vi "examen2_1.vi"() -> ()   [LabVIEW 2020]
panel:
  out "String":string
  in  "Tab Control":enum32{"servicio", "mantenimiento"}(tab)=enum."mantenimiento"
  in  "COFFEE":bool
  in  "COLD DRINK":bool
  in  "CANDIES":bool
  in  "SNACKS":bool
  in  "$20":bool
  in  "$10":bool
  out "$ INGRESADA":dbl
  in  "INICILIZAR":bool
  out "$ DEVOLVER":dbl
  out "$ FALTANTE":dbl
  in  "CANCELAR":bool
  out "v. $10":dbl
  out "v. $20":dbl
  in  "in. snack":dbl=4.0
  in  "in. coffee":dbl=4.0
  in  "in. cold drink":dbl=4.0
  in  "in. candies":dbl=4.0
  # "VALOR IN $ 10"
  # "VALOR IN $ 20"
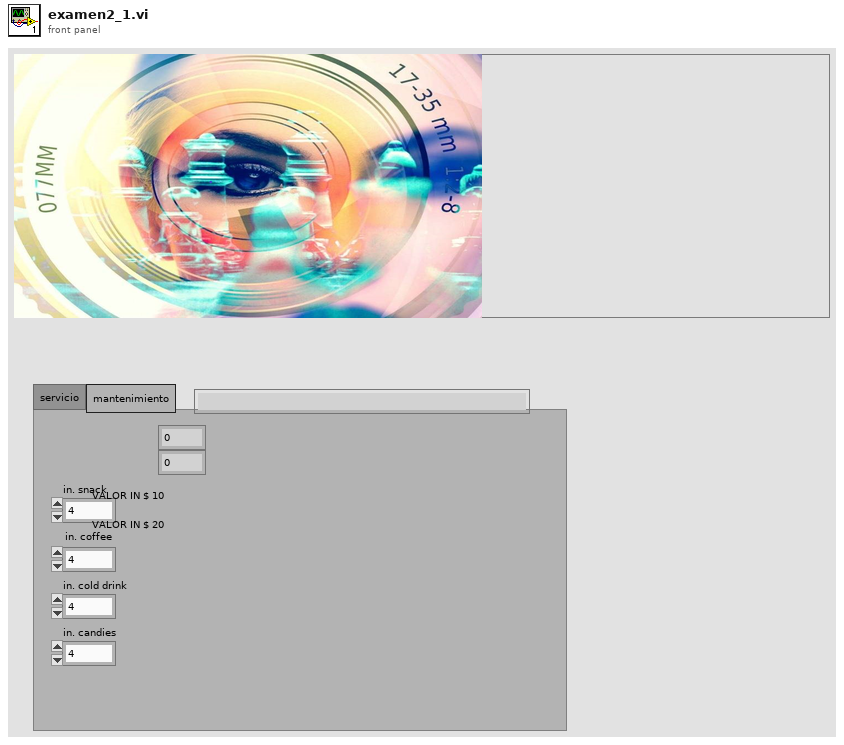
[diagram p1: front panel]
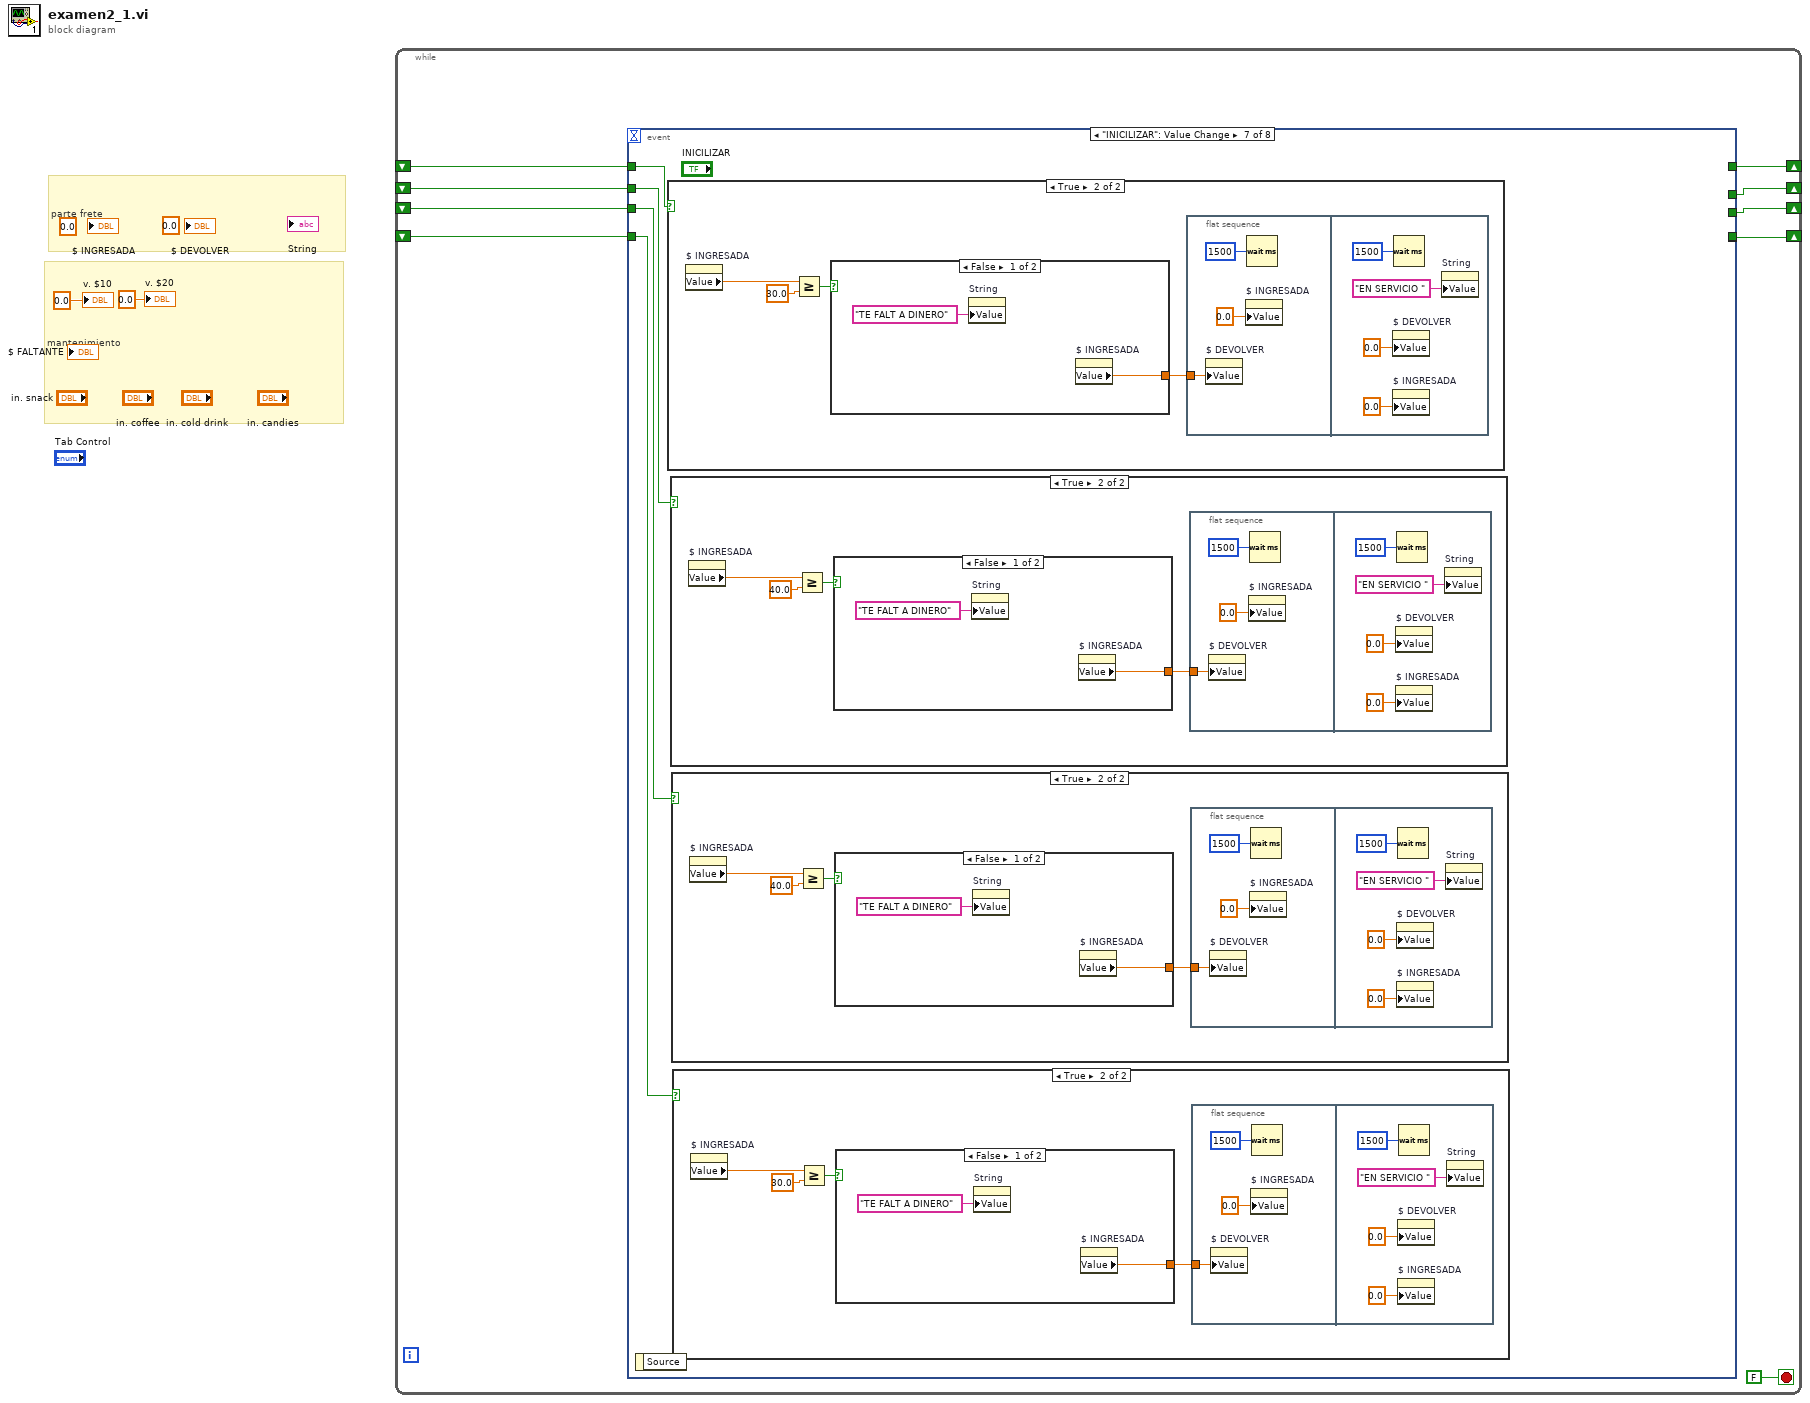
[diagram p0: block diagram]
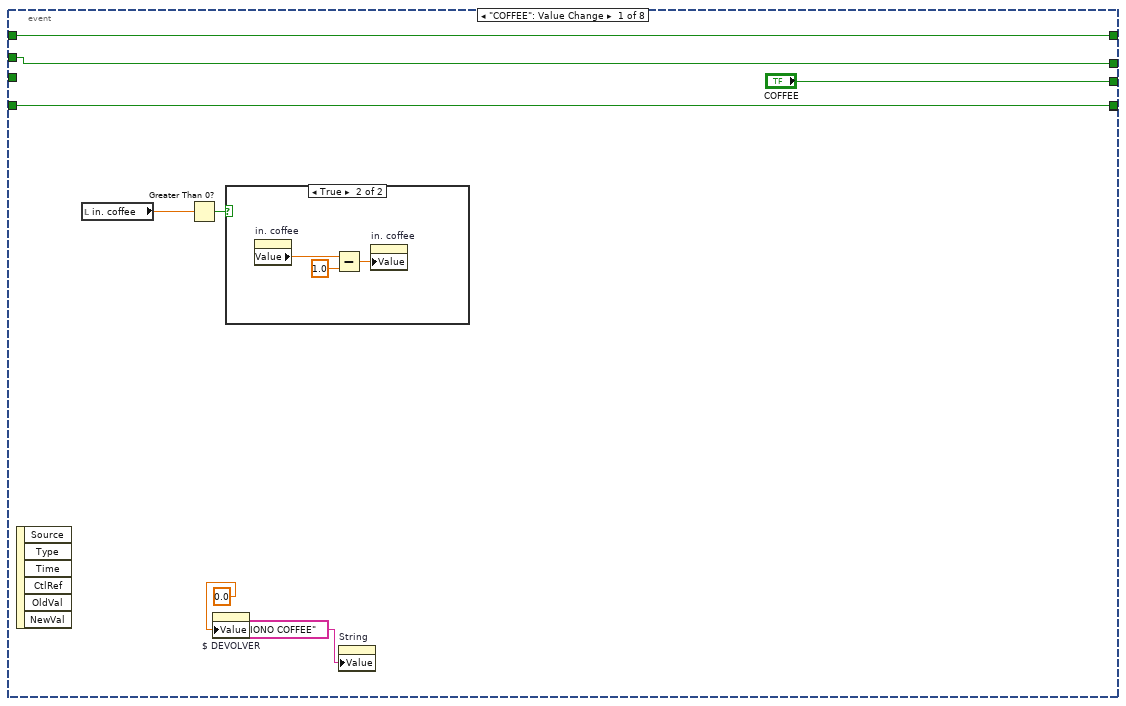
[diagram p2: hidden frame]
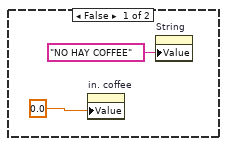
[diagram p3: hidden frame]
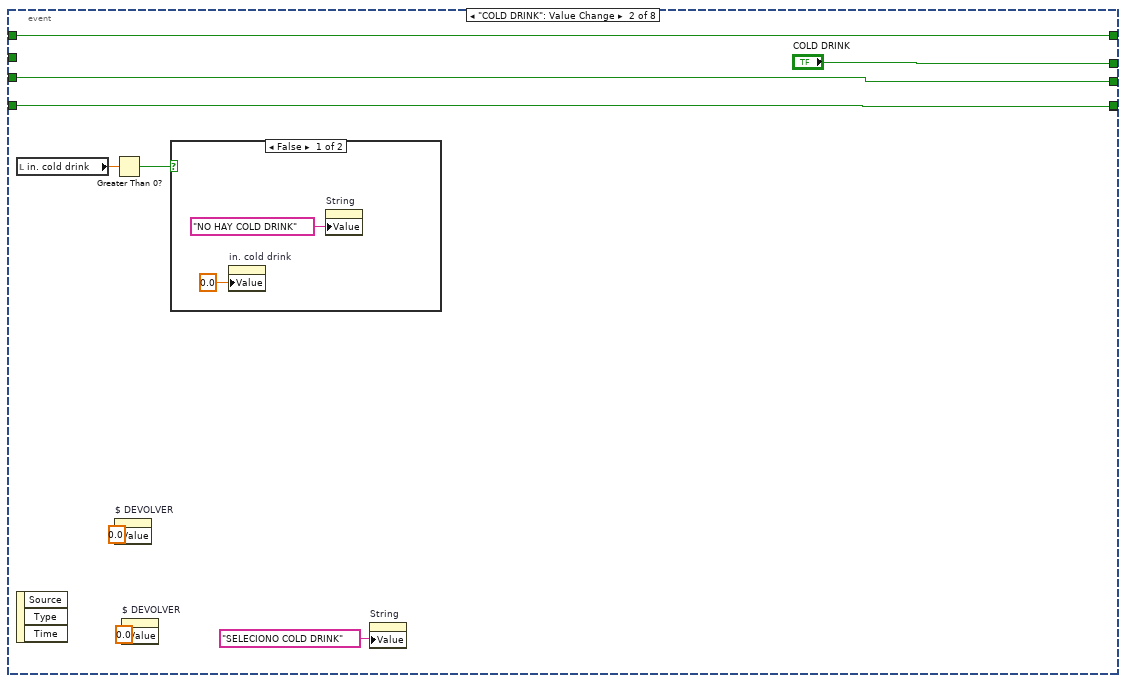
[diagram p4: hidden frame]
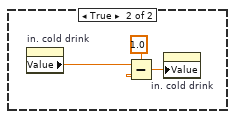
[diagram p5: hidden frame]
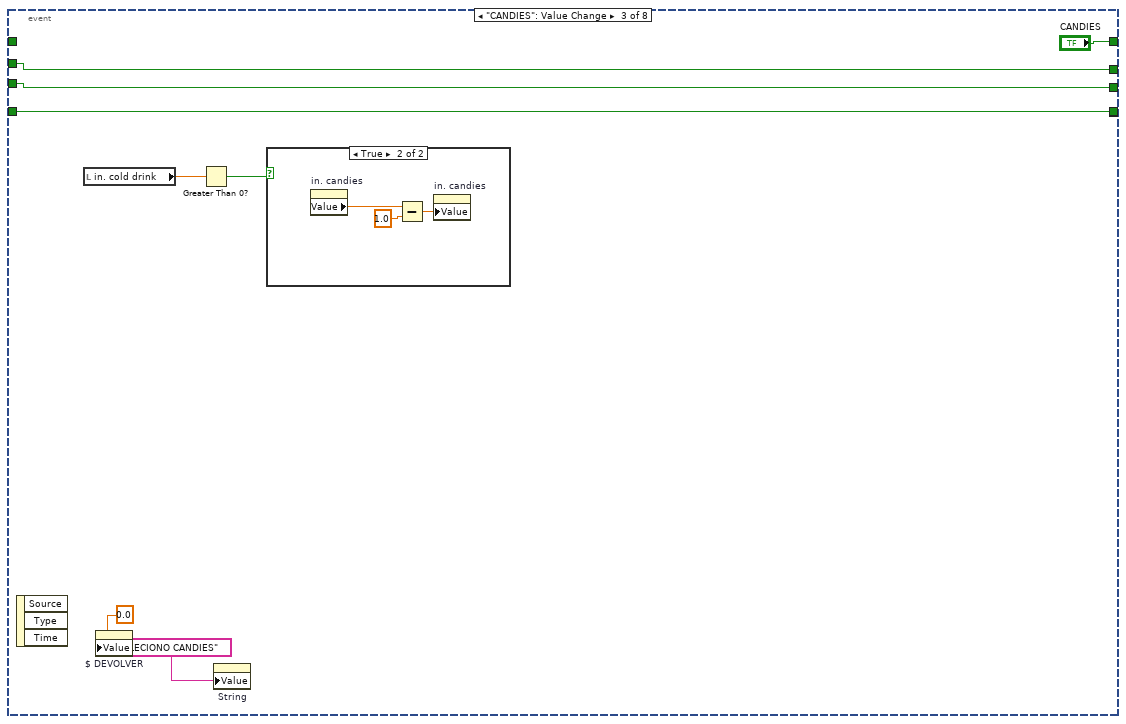
[diagram p6: hidden frame]
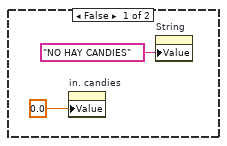
[diagram p7: hidden frame]
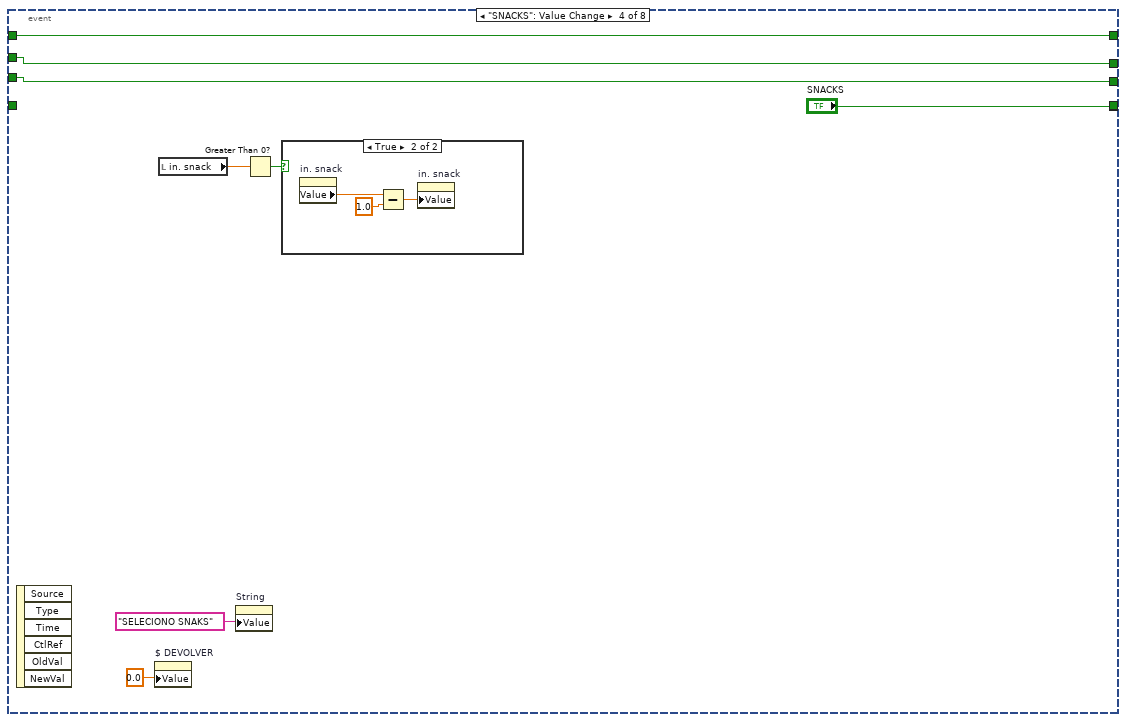
[diagram p8: hidden frame]
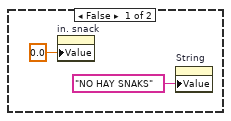
[diagram p9: hidden frame]
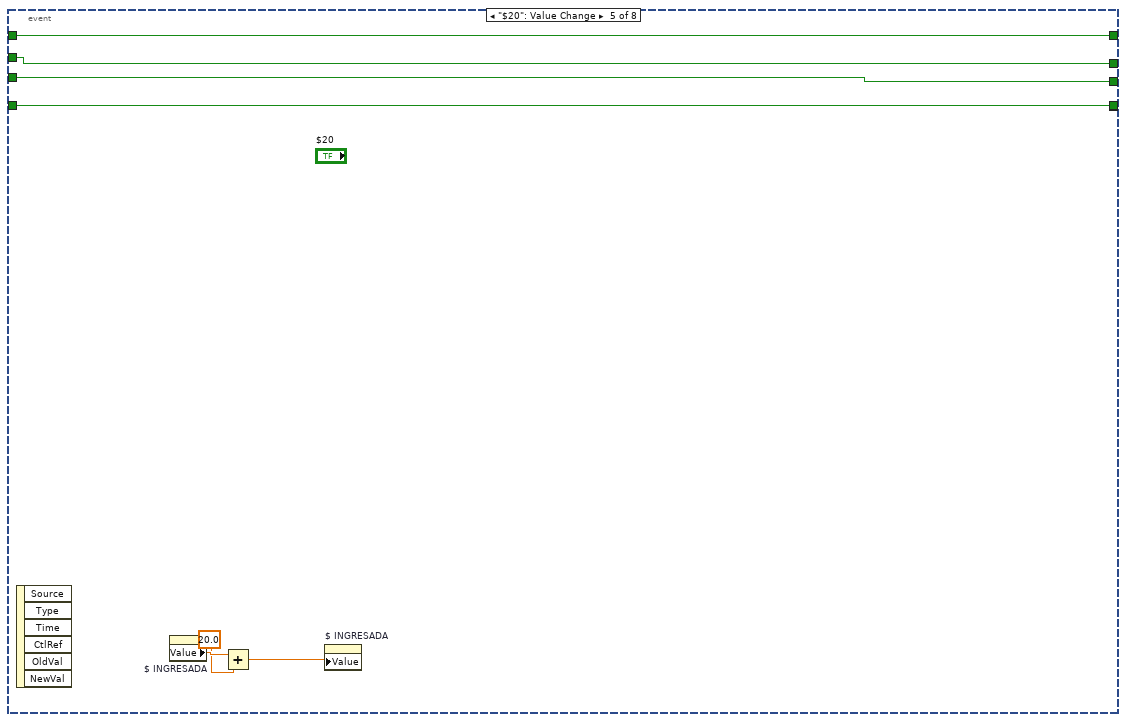
[diagram p10: hidden frame]
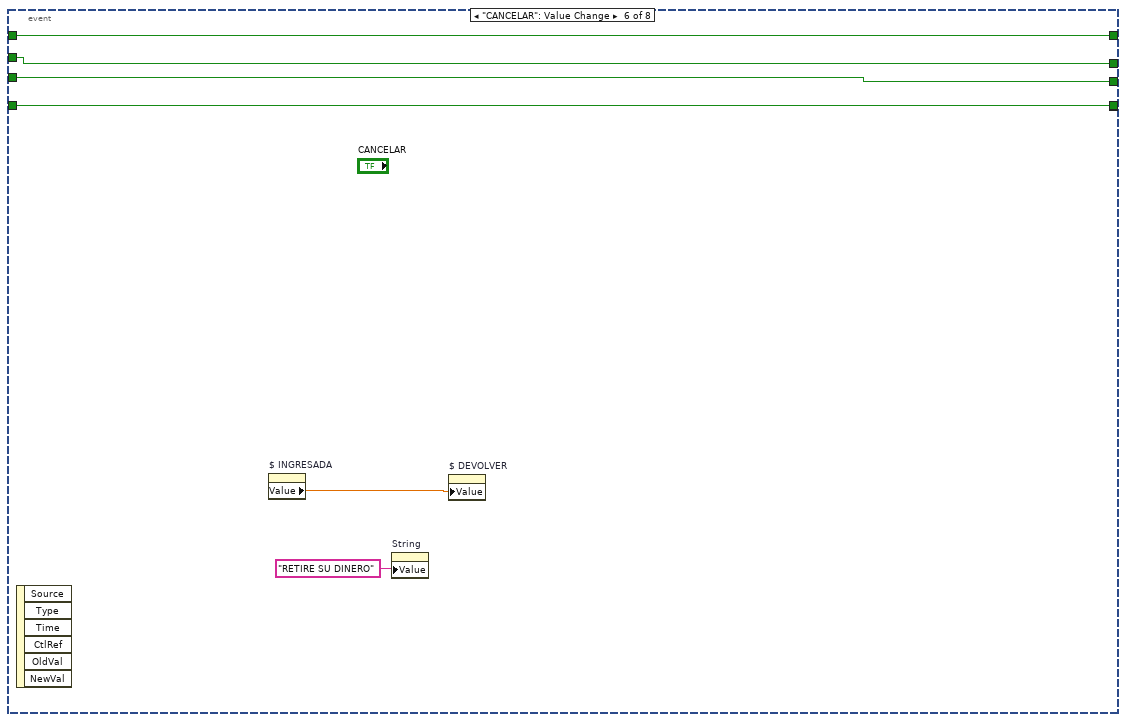
[diagram p11: hidden frame]
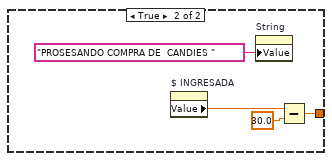
[diagram p13: hidden frame]
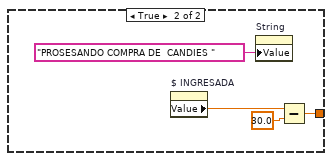
[diagram p15: hidden frame]
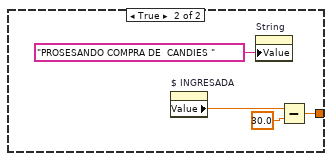
[diagram p17: hidden frame]
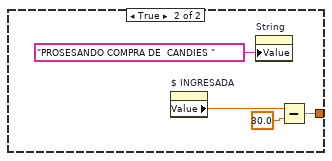
[diagram p19: hidden frame]
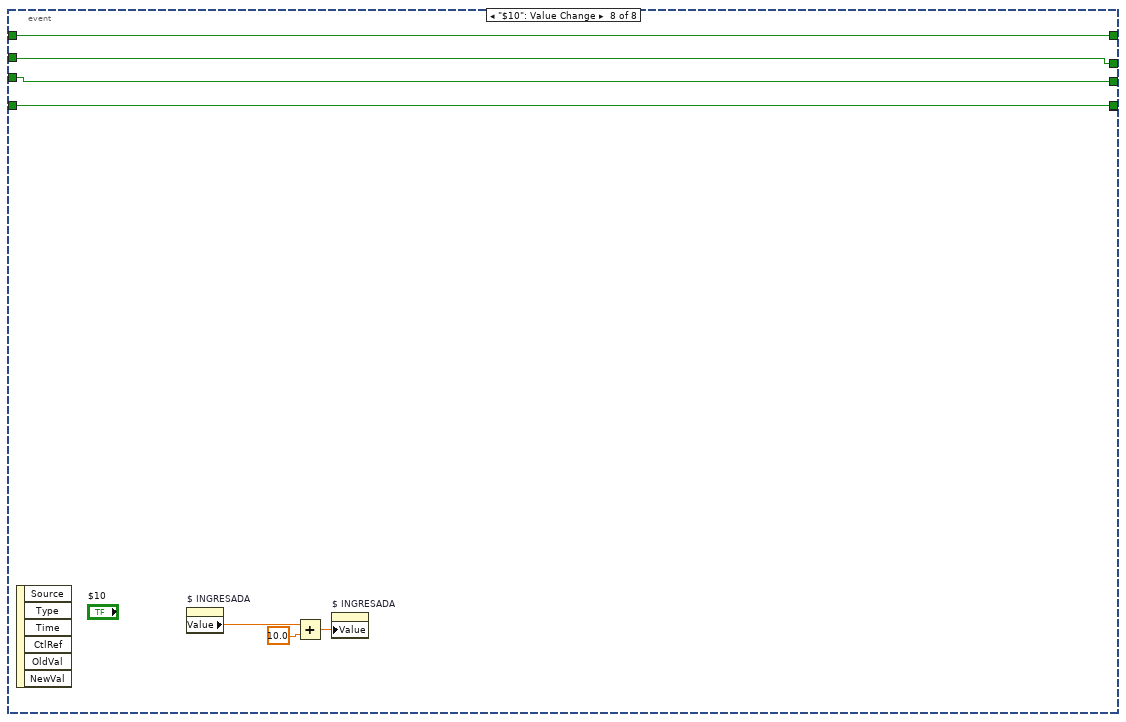
[diagram p20: hidden frame]
diagram:
  # "parte frete"
  # "mantenimiento"
  n1 = while {
    shift-right: [w12] -> _
    shift-left: _ -> [w11]
    shift-right: [w10] -> _
    shift-left: _ -> [w9]
    shift-right: [w8] -> _
    shift-left: _ -> [w7]
    shift-right: [w6] -> _
    shift-left: _ -> [w5]
    stop <- FALSE stop-if-true
    n2 = event shown="[6] \"INICILIZAR\": Value Change" {
      selector: _ -> [_ _ _ _ _ _ _ _]
      dyn-events: _ -> [_ _ _ _ _ _ _ _]
      timeout: _ -> [_ _ _ _ _ _ _ _]
      tunnel: [w19 "COLD DRINK" w46 w59 w70 w76 _ w155] -> w12
      tunnel: w11 -> [w19 _ w46 w59 w70 w76 w80 w155]
      tunnel: [w16 w29 "CANDIES" w58 w69 _ _ w154] -> w10
      tunnel: w9 -> [w16 w29 _ w58 w69 w77 w83 w154]
      tunnel: ["COFFEE" w28 w42 w57 w68 w74 _ w153] -> w8
      tunnel: w7 -> [_ w28 w42 w57 w68 w74 w81 w153]
      tunnel: [w14 w27 w41 "SNACKS" w67 _ _ w152] -> w6
      tunnel: w5 -> [w14 w27 w41 _ w67 w75 w82 w152]
      tunnel: [_ _ _ _ _ w77 _ _] -> _
      tunnel: [_ _ _ _ _ w75 _ _] -> _
      event "COFFEE": Value Change {
        n3 = event-data() -> ()  [unwired: 1 in, 6 out]
        n4 = local read "in. coffee"() -> (w18:dbl)
        n5 = Greater Than 0?(x=w18) -> (x > 0?=w17:bool)
        n6 = property on="$ DEVOLVER" class="DigNum (strict)"("Value"=0.0 ("$ DEVOLVER")) -> ()  [unwired: 2 in, 2 out]
        n7 = case shown="True" w17 {
          frame False {
            n8 = property on="in. coffee" class="DigNum (strict)"("Value"=0.0 ("in. cold drink")) -> ()  [unwired: 2 in, 2 out]
            n9 = property on="String" class="Str"("Value"="NO HAY COFFEE" ("String")) -> ()  [unwired: 2 in, 2 out]
          }
          frame True {
            n10 = property on="in. coffee" class="DigNum (strict)"() -> ("Value"=w26:dbl)  [unwired: 2 in, 2 out]
            n11 = Subtract(x=w26, y=1.0) -> (x-y=w25:dbl)
            n12 = property on="in. coffee" class="DigNum (strict)"("Value"=w25) -> ()  [unwired: 2 in, 2 out]
          }
        }
        n13 = property on="String" class="Str"("Value"="SELECIONO COFFEE" ("String")) -> ()  [unwired: 2 in, 2 out]
      }
      event "COLD DRINK": Value Change {
        n14 = local read "in. cold drink"() -> (w33:dbl)
        n15 = event-data() -> ()  [unwired: 1 in, 3 out]
        n16 = Greater Than 0?(x=w33) -> (x > 0?=w32:bool)
        n17 = property on="$ DEVOLVER" class="DigNum (strict)"("Value"=0.0 ("$ DEVOLVER")) -> ()  [unwired: 2 in, 2 out]
        n18 = property on="$ DEVOLVER" class="DigNum (strict)"("Value"=0.0 ("$ DEVOLVER")) -> ()  [unwired: 2 in, 2 out]
        n19 = case shown="False" w32 {
          frame False {
            n20 = property on="in. cold drink" class="DigNum (strict)"("Value"=0.0 ("in. cold drink")) -> ()  [unwired: 2 in, 2 out]
            n21 = property on="String" class="Str"("Value"="NO HAY COLD DRINK" ("String")) -> ()  [unwired: 2 in, 2 out]
          }
          frame True {
            n22 = property on="in. cold drink" class="DigNum (strict)"() -> ("Value"=w40:dbl)  [unwired: 2 in, 2 out]
            n23 = Subtract(x=w40, y=1.0) -> (x-y=w39:dbl)
            n24 = property on="in. cold drink" class="DigNum (strict)"("Value"=w39) -> ()  [unwired: 2 in, 2 out]
          }
        }
        n25 = property on="String" class="Str"("Value"="SELECIONO COLD DRINK" ("String")) -> ()  [unwired: 2 in, 2 out]
      }
      event "CANDIES": Value Change {
        n26 = event-data() -> ()  [unwired: 1 in, 3 out]
        n27 = local read "in. cold drink"() -> (w45:dbl)
        n28 = property on="$ DEVOLVER" class="DigNum (strict)"("Value"=0.0 ("$ DEVOLVER")) -> ()  [unwired: 2 in, 2 out]
        n29 = Greater Than 0?(x=w45) -> (x > 0?=w44:bool)
        n30 = property on="String" class="Str"("Value"="SELECIONO CANDIES" ("String")) -> ()  [unwired: 2 in, 2 out]
        n31 = case shown="True" w44 {
          frame False {
            n32 = property on="in. candies" class="DigNum (strict)"("Value"=0.0 ("in. cold drink")) -> ()  [unwired: 2 in, 2 out]
            n33 = property on="String" class="Str"("Value"="NO HAY CANDIES" ("String")) -> ()  [unwired: 2 in, 2 out]
          }
          frame True {
            n34 = property on="in. candies" class="DigNum (strict)"() -> ("Value"=w53:dbl)  [unwired: 2 in, 2 out]
            n35 = Subtract(x=w53, y=1.0) -> (x-y=w52:dbl)
            n36 = property on="in. candies" class="DigNum (strict)"("Value"=w52) -> ()  [unwired: 2 in, 2 out]
          }
        }
      }
      event "SNACKS": Value Change {
        n37 = event-data() -> ()  [unwired: 1 in, 6 out]
        n38 = property on="$ DEVOLVER" class="DigNum (strict)"("Value"=0.0 ("$ DEVOLVER")) -> ()  [unwired: 2 in, 2 out]
        n39 = local read "in. snack"() -> (w55:dbl)
        n40 = property on="String" class="Str"("Value"="SELECIONO SNAKS" ("String")) -> ()  [unwired: 2 in, 2 out]
        n41 = Greater Than 0?(x=w55) -> (x > 0?=w54:bool)
        n42 = case shown="True" w54 {
          frame False {
            n43 = property on="in. snack" class="DigNum (strict)"("Value"=0.0 ("in. cold drink")) -> ()  [unwired: 2 in, 2 out]
            n44 = property on="String" class="Str"("Value"="NO HAY SNAKS" ("String")) -> ()  [unwired: 2 in, 2 out]
          }
          frame True {
            n45 = property on="in. snack" class="DigNum (strict)"() -> ("Value"=w65:dbl)  [unwired: 2 in, 2 out]
            n46 = Subtract(x=w65, y=1.0) -> (x-y=w66:dbl)
            n47 = property on="in. snack" class="DigNum (strict)"("Value"=w66) -> ()  [unwired: 2 in, 2 out]
          }
        }
      }
      event "$20": Value Change {
        n48 = event-data() -> ()  [unwired: 1 in, 6 out]
        n49 = property on="$ INGRESADA" class="DigNum (strict)"() -> ("Value"=w73:dbl)  [unwired: 2 in, 2 out]
        n50 = Add(x=w73, y=20.0) -> (x+y=w71:dbl)
        n51 = property on="$ INGRESADA" class="DigNum (strict)"("Value"=w71) -> ()  [unwired: 2 in, 2 out]
      }
      event "CANCELAR": Value Change {
        n52 = event-data() -> ()  [unwired: 1 in, 6 out]
        n53 = property on="$ INGRESADA" class="DigNum (strict)"() -> ("Value"=w79:dbl)  [unwired: 2 in, 2 out]
        n54 = property on="String" class="Str"("Value"="RETIRE SU DINERO" ("String")) -> ()  [unwired: 2 in, 2 out]
        n55 = property on="$ DEVOLVER" class="DigNum (strict)"("Value"=w79) -> ()  [unwired: 2 in, 2 out]
      }
      event "INICILIZAR": Value Change {
        n56 = event-data() -> ()  [unwired: 1 in, 1 out]
        n57 = case shown="True" w83 {
          frame False {
          }
          frame True {
            n58 = property on="$ INGRESADA" class="DigNum (strict)"() -> ("Value"=w138:dbl)  [unwired: 2 in, 2 out]
            n59 = Greater Or Equal?(x=w138, y=30.0) -> (x >= y?=w136:bool)
            n60 = case shown="False" w136 {
              tunnel: [w147 w149] -> w135
              frame False {
                n61 = property on="String" class="Str"("Value"="TE FALT A DINERO" ("String")) -> ()  [unwired: 2 in, 2 out]
                n62 = property on="$ INGRESADA" class="DigNum (strict)"() -> ("Value"=w147:dbl)  [unwired: 2 in, 2 out]
              }
              frame True {
                n63 = property on="$ INGRESADA" class="DigNum (strict)"() -> ("Value"=w151:dbl)  [unwired: 2 in, 2 out]
                n64 = property on="String" class="Str"("Value"="PROSESANDO COMPRA DE  CANDIES " ("String")) -> ()  [unwired: 2 in, 2 out]
                n65 = Subtract(x=w151, y=30.0) -> (x-y=w149:dbl)
              }
            }
            n66 = flat-sequence {
              tunnel: w135 -> [w141]
              frame #0 {
                n67 = property on="$ DEVOLVER" class="DigNum (strict)"("Value"=w141) -> ()  [unwired: 2 in, 2 out]
                n68 = property on="$ INGRESADA" class="DigNum (strict)"("Value"=0.0 ("$ INGRESADA")) -> ()  [unwired: 2 in, 2 out]
                n69 = Wait (ms)(milliseconds to wait=u32 1500) -> ()  [unwired: 1 out]
              }
              frame #1 {
                n70 = property on="$ DEVOLVER" class="DigNum (strict)"("Value"=0.0 ("$ DEVOLVER")) -> ()  [unwired: 2 in, 2 out]
                n71 = property on="$ INGRESADA" class="DigNum (strict)"("Value"=0.0 ("$ INGRESADA")) -> ()  [unwired: 2 in, 2 out]
                n72 = Wait (ms)(milliseconds to wait=u32 1500) -> ()  [unwired: 1 out]
                n73 = property on="String" class="Str"("Value"="EN SERVICIO " ("String")) -> ()  [unwired: 2 in, 2 out]
              }
            }
          }
        }
        n74 = case shown="True" w80 {
          frame False {
          }
          frame True {
            n75 = property on="$ INGRESADA" class="DigNum (strict)"() -> ("Value"=w121:dbl)  [unwired: 2 in, 2 out]
            n76 = Greater Or Equal?(x=w121, y=40.0) -> (x >= y?=w119:bool)
            n77 = case shown="False" w119 {
              tunnel: [w130 w132] -> w118
              frame False {
                n78 = property on="String" class="Str"("Value"="TE FALT A DINERO" ("String")) -> ()  [unwired: 2 in, 2 out]
                n79 = property on="$ INGRESADA" class="DigNum (strict)"() -> ("Value"=w130:dbl)  [unwired: 2 in, 2 out]
              }
              frame True {
                n80 = property on="$ INGRESADA" class="DigNum (strict)"() -> ("Value"=w134:dbl)  [unwired: 2 in, 2 out]
                n81 = property on="String" class="Str"("Value"="PROSESANDO COMPRA DE  CANDIES " ("String")) -> ()  [unwired: 2 in, 2 out]
                n82 = Subtract(x=w134, y=30.0) -> (x-y=w132:dbl)
              }
            }
            n83 = flat-sequence {
              tunnel: w118 -> [w124]
              frame #0 {
                n84 = property on="$ DEVOLVER" class="DigNum (strict)"("Value"=w124) -> ()  [unwired: 2 in, 2 out]
                n85 = property on="$ INGRESADA" class="DigNum (strict)"("Value"=0.0 ("$ INGRESADA")) -> ()  [unwired: 2 in, 2 out]
                n86 = Wait (ms)(milliseconds to wait=u32 1500) -> ()  [unwired: 1 out]
              }
              frame #1 {
                n87 = property on="$ DEVOLVER" class="DigNum (strict)"("Value"=0.0 ("$ DEVOLVER")) -> ()  [unwired: 2 in, 2 out]
                n88 = property on="$ INGRESADA" class="DigNum (strict)"("Value"=0.0 ("$ INGRESADA")) -> ()  [unwired: 2 in, 2 out]
                n89 = Wait (ms)(milliseconds to wait=u32 1500) -> ()  [unwired: 1 out]
                n90 = property on="String" class="Str"("Value"="EN SERVICIO " ("String")) -> ()  [unwired: 2 in, 2 out]
              }
            }
          }
        }
        n91 = case shown="True" w81 {
          frame False {
          }
          frame True {
            n92 = property on="$ INGRESADA" class="DigNum (strict)"() -> ("Value"=w104:dbl)  [unwired: 2 in, 2 out]
            n93 = Greater Or Equal?(x=w104, y=40.0) -> (x >= y?=w102:bool)
            n94 = case shown="False" w102 {
              tunnel: [w113 w115] -> w101
              frame False {
                n95 = property on="String" class="Str"("Value"="TE FALT A DINERO" ("String")) -> ()  [unwired: 2 in, 2 out]
                n96 = property on="$ INGRESADA" class="DigNum (strict)"() -> ("Value"=w113:dbl)  [unwired: 2 in, 2 out]
              }
              frame True {
                n97 = property on="$ INGRESADA" class="DigNum (strict)"() -> ("Value"=w117:dbl)  [unwired: 2 in, 2 out]
                n98 = property on="String" class="Str"("Value"="PROSESANDO COMPRA DE  CANDIES " ("String")) -> ()  [unwired: 2 in, 2 out]
                n99 = Subtract(x=w117, y=30.0) -> (x-y=w115:dbl)
              }
            }
            n100 = flat-sequence {
              tunnel: w101 -> [w107]
              frame #0 {
                n101 = property on="$ DEVOLVER" class="DigNum (strict)"("Value"=w107) -> ()  [unwired: 2 in, 2 out]
                n102 = property on="$ INGRESADA" class="DigNum (strict)"("Value"=0.0 ("$ INGRESADA")) -> ()  [unwired: 2 in, 2 out]
                n103 = Wait (ms)(milliseconds to wait=u32 1500) -> ()  [unwired: 1 out]
              }
              frame #1 {
                n104 = property on="$ DEVOLVER" class="DigNum (strict)"("Value"=0.0 ("$ DEVOLVER")) -> ()  [unwired: 2 in, 2 out]
                n105 = property on="$ INGRESADA" class="DigNum (strict)"("Value"=0.0 ("$ INGRESADA")) -> ()  [unwired: 2 in, 2 out]
                n106 = Wait (ms)(milliseconds to wait=u32 1500) -> ()  [unwired: 1 out]
                n107 = property on="String" class="Str"("Value"="EN SERVICIO " ("String")) -> ()  [unwired: 2 in, 2 out]
              }
            }
          }
        }
        n108 = case shown="True" w82 {
          frame False {
          }
          frame True {
            n109 = property on="$ INGRESADA" class="DigNum (strict)"() -> ("Value"=w87:dbl)  [unwired: 2 in, 2 out]
            n110 = Greater Or Equal?(x=w87, y=30.0) -> (x >= y?=w85:bool)
            n111 = case shown="False" w85 {
              tunnel: [w96 w98] -> w84
              frame False {
                n112 = property on="String" class="Str"("Value"="TE FALT A DINERO" ("String")) -> ()  [unwired: 2 in, 2 out]
                n113 = property on="$ INGRESADA" class="DigNum (strict)"() -> ("Value"=w96:dbl)  [unwired: 2 in, 2 out]
              }
              frame True {
                n114 = property on="$ INGRESADA" class="DigNum (strict)"() -> ("Value"=w100:dbl)  [unwired: 2 in, 2 out]
                n115 = property on="String" class="Str"("Value"="PROSESANDO COMPRA DE  CANDIES " ("String")) -> ()  [unwired: 2 in, 2 out]
                n116 = Subtract(x=w100, y=30.0) -> (x-y=w98:dbl)
              }
            }
            n117 = flat-sequence {
              tunnel: w84 -> [w90]
              frame #0 {
                n118 = property on="$ DEVOLVER" class="DigNum (strict)"("Value"=w90) -> ()  [unwired: 2 in, 2 out]
                n119 = property on="$ INGRESADA" class="DigNum (strict)"("Value"=0.0 ("$ INGRESADA")) -> ()  [unwired: 2 in, 2 out]
                n120 = Wait (ms)(milliseconds to wait=u32 1500) -> ()  [unwired: 1 out]
              }
              frame #1 {
                n121 = property on="$ DEVOLVER" class="DigNum (strict)"("Value"=0.0 ("$ DEVOLVER")) -> ()  [unwired: 2 in, 2 out]
                n122 = property on="$ INGRESADA" class="DigNum (strict)"("Value"=0.0 ("$ INGRESADA")) -> ()  [unwired: 2 in, 2 out]
                n123 = Wait (ms)(milliseconds to wait=u32 1500) -> ()  [unwired: 1 out]
                n124 = property on="String" class="Str"("Value"="EN SERVICIO " ("String")) -> ()  [unwired: 2 in, 2 out]
              }
            }
          }
        }
      }
      event "$10": Value Change {
        n125 = event-data() -> ()  [unwired: 1 in, 6 out]
        n126 = property on="$ INGRESADA" class="DigNum (strict)"() -> ("Value"=w156:dbl)  [unwired: 2 in, 2 out]
        n127 = Add(x=w156, y=10.0) -> (x+y=w157:dbl)
        n128 = property on="$ INGRESADA" class="DigNum (strict)"("Value"=w157) -> ()  [unwired: 2 in, 2 out]
      }
    }
  }
  "v. $20" <- 0.0 ("v. $20")
  "$ INGRESADA" <- 0.0 ("$ INGRESADA")
  "v. $10" <- 0.0 ("v. $10")
  "$ DEVOLVER" <- 0.0 ("$ DEVOLVER")
